vi "quantile_transform.vi"(8 "error in":errorcluster caption="entrée d'erreur", 9 "X":string[][](array[string]), 10 "Type X":T1(ring), 11 "quantile_transform":T3={"axis"=0, "n_quantiles"=1000, "output_distribution"="uniform", "ignore_implicit_zeros"=FALSE, "subsample"=100000.0, "random_state"=-1, "copy"=TRUE} {"random_state" min=-1}) -> (0 "error out":errorcluster caption="sortie d'erreur", 3 "Data":T2)   [LabVIEW 2020]
doc: "Transform features using quantiles information.\n\nThis method transforms the features to follow a uniform or a normal distribution. Therefore, for a given feature, this transformation tends to spread out the most frequent values. It also reduces the impact of (marginal) outliers: this is therefore a robust preprocessing scheme.\n\nThe transformation is applied on each feature independently. First an estimate of the cumulative distribution function of a feature is used to map the original values to a uniform distribution. The obtained values are then mapped to the desired output distribution using the associated quantile function. Features values of new/unseen data that fall below or above the fitted range will be mapped to the bounds of the output distribution. Note that this transform is non-linear. It may distort linear correlations between variables measured at the same scale but renders variables measured at different scales more directly comparable.\n\n\nParameters :\n\n- X : array-like, sparse matrix\nThe data to transform.\n\n- axis : int, (default=0)\nAxis used to compute the means and standard deviations along. If 0, transform each feature, otherwise (if 1) transform each sample.\n\n- n_quantiles : int, optional (default=1000 or n_samples)\nNumber of quantiles to be computed. It corresponds to the number of landmarks used to discretize the cumulative distribution function. If n_quantiles is larger than the number of samples, n_quantiles is set to the number of samples as a larger number of quantiles does not give a better approximation of the cumulative distribution function estimator.\n\n- output_distribution : str, optional (default=’uniform’)\nMarginal distribution for the transformed data. The choices are ‘uniform’ (default) or ‘normal’.\n\n- ignore_implicit_zeros : bool, optional (default=False)\nOnly applies to sparse matrices. If True, the sparse entries of the matrix are discarded to compute the quantile statistics. If False, these entries are treated as zeros.\n\n- subsample : int, optional (default=1e5)\nMaximum number of samples used to estimate the quantiles for computational efficiency. Note that the subsampling procedure may differ for value-identical sparse and dense matrices.\n\n- random_state : int, RandomState instance or None, optional (default=None=-1)\nDetermines random number generation for subsampling and smoothing noise. Please see subsample for more details. Pass an int for reproducible results across multiple function calls. See Glossary\n\n- copy : boolean, optional, (default=True)\nSet to False to perform inplace transformation and avoid a copy (if the input is already a numpy array). If True, a copy of X is transformed, leaving the original X unchanged\n\n\nReturns : \n\n- Xt : ndarray or sparse matrix, shape (n_samples, n_features)\nThe transformed data."
uses:
  quantile_transform.lvclass
panel:
  out "quantile_transform.lvclass":refnum<class "quantile_transform.lvclass">
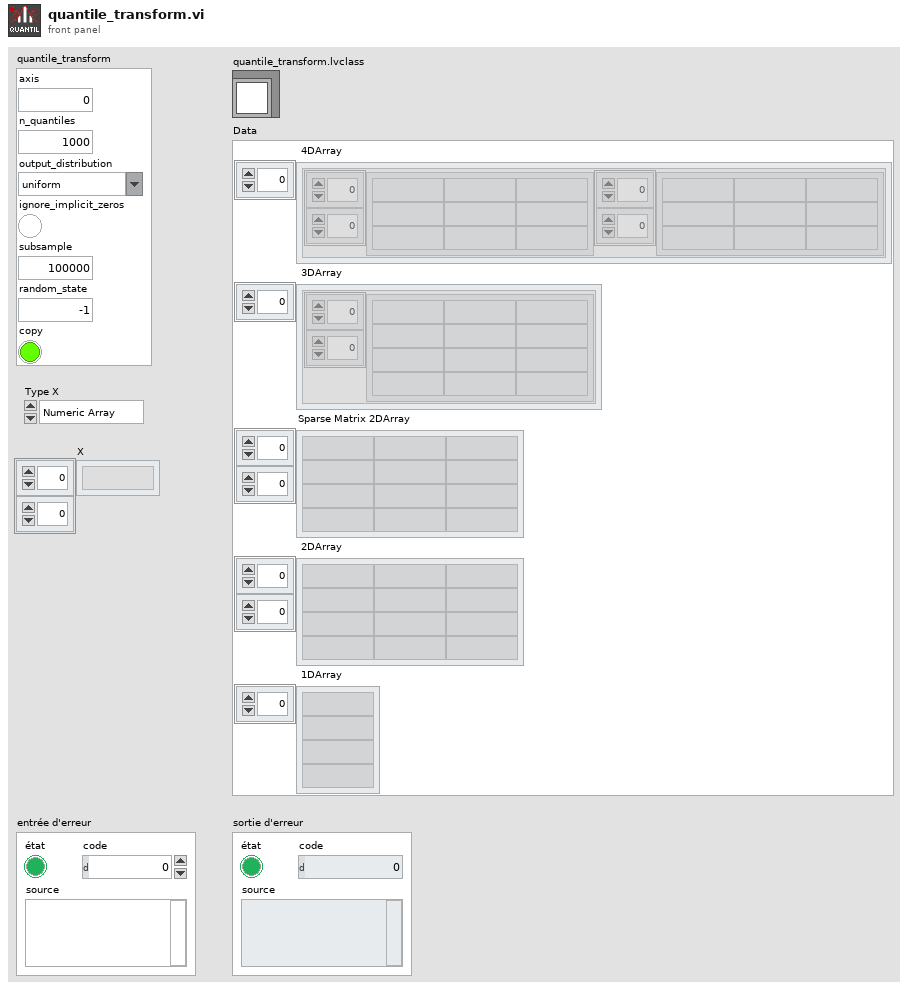
[diagram p1: front panel]
types:
  T1 = enum16{"Numeric Array", "String Array", "Sparse"}
  T2 = cluster{" 4DArray":cluster{"1":string[][], "2":string[][]}[], " 3DArray":cluster{"Tableau":string[][]}[], "Sparse Matrix 2DArray":string[][], " 2DArray":string[][], " 1DArray":string[]}
  T3 = cluster{"axis":i32, "n_quantiles":i32, "output_distribution":string, "ignore_implicit_zeros":bool, "subsample":dbl, "random_state":i32, "copy":bool}
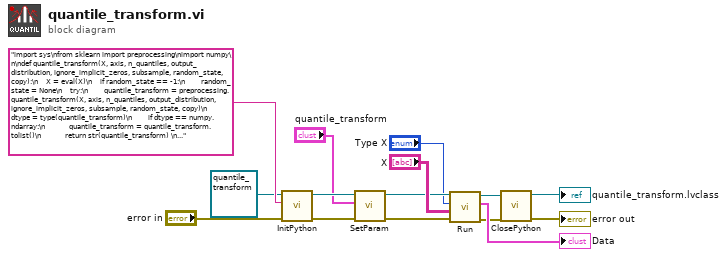
[diagram p0: block diagram]
diagram:
  n1 = call-dynamic "InitPython.vi"("error in (no error)"="error in", "Python Instruction"="import sys\nfrom sklearn import preprocessing\nimport numpy\n\ndef quantile_transform(X, axis, n_quantiles, output_distribution, ignore_implicit_zeros, subsample, random_state, copy):\n    X = eval(X)\n    if random_state == -1:\n        random_state = None\n    try:\n        quantile_transform = preprocessing.quantile_transform(X, axis, n_quantiles, output_distribution, ignore_implicit_zeros, subsample, random_state, copy)\n        dtype = type(quantile_transform)\n        if dtype == numpy.ndarray:\n            quantile_transform = quantile_transform.tolist()\n            return str(quantile_transform) \n        else:\n            Mat = quantile_transform.tocoo()\n            return str(list(zip(Mat.row, Mat.col, Mat.data)))\n    except:\n        erreur = sys.exc_info()\n        typerr = u\"%s\" % (erreur[0])\n        typerr = typerr[typerr.find(\"'\")+1:typerr.rfind(\"'\")]\n        msgerr = u\"%s\" % (erreur[1])\n        message = str('/!\\\\ {0} : {1}'. format(typerr,msgerr))\n        return message", "Scikit-learn en entrée"=refnum<class "quantile_transform.lvclass"> refnum ("quantile_transform.lvclass")) -> ("error out"=w10:errorcluster, "Scikit-learn en sortie"=w11:refnum<class "quantile_transform.lvclass">)  [unwired: 7 in]
  n2 = call-dynamic "SetParam.vi"("error in (no error)"=w10, "quantile_transform"="quantile_transform", "quantile_transform.lvclass"=w11) -> ("error out"=w3:errorcluster, "quantile_transform.lvclass"=w4:refnum<class "quantile_transform.lvclass">)  [unwired: 7 in]
  n3 = call-dynamic "Run.vi"("error in (no error)"=w3, "X"="X", "Type X"="Type X", "quantile_transform.lvclass"=w4) -> ("error out"=w6:errorcluster, "Data"=→"Data":T2, "quantile_transform.lvclass"=w8:refnum<class "quantile_transform.lvclass">)  [unwired: 5 in]
  n4 = call-dynamic "ClosePython.vi"("error in (no error)"=w6, "Scikit-learn en entrée"=w8) -> ("error out"=→"error out":errorcluster, "Scikit-learn en sortie"=→"quantile_transform.lvclass":refnum<class "quantile_transform.lvclass">)  [unwired: 8 in]
